vi "Find Next Control Word Address.vi"(7 "Half Step? (F)":bool, 11 "Starting Address":u16 format="%04x") -> (3 "0xHHHX Address":u16 format="%04x")   [LabVIEW 2020, in "BCI-1553 API.lvlib"]
doc: "Take in an address and find the next base 8 or base 16 address. This VI will normally return the next base 16 whole address. If a half step is selected, the next whole base 8 address is returned. \n\nA whole address is such that when divided by the base, it produces no remainder."
uses:
  BCI-1553 API.lvlib
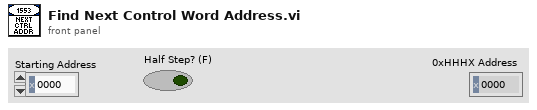
[diagram p1: front panel]
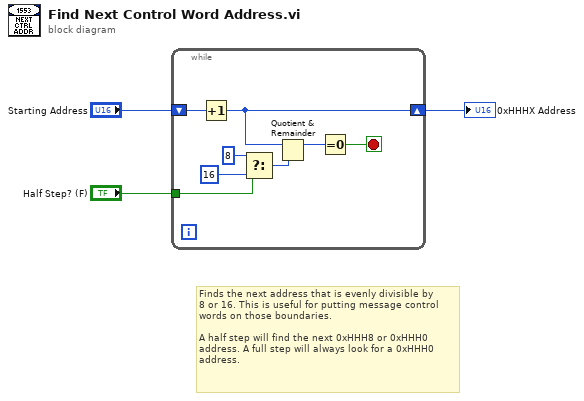
[diagram p0: block diagram]
diagram:
  # "Finds the next address that is evenly divisible by\n8 or 16. This is useful for putting message control\nwords on those boundaries.\n\nA half step will find the next 0xHHH8 or 0xHHH0\naddress. A full step will always look for a 0xHHH0\naddress."
  n1 = while {
    shift-right: [w10] -> w2
    shift-left: "Starting Address" -> [w11]
    tunnel: "Half Step? (F)" -> [w4]
    stop <- w8 stop-if-true
    n2 = Increment(x=w11) -> (x+1=w10:u16)
    n3 = Select(t=u16 8 ("y"), s=w4, f=u16 16 ("y")) -> (s? t:f=w5:u16)
    n4 = Quotient & Remainder(x=w10, y=w5) -> (x-y*floor(x/y)=w9:u16)  [unwired: 1 out]
    n5 = Equal To 0?(x=w9) -> (x = 0?=w8:bool)
  }
  "0xHHHX Address" <- w2
